vi "oa_Config Time or RPM Segment.vi"(0 "time segment":T2 {"step (s)" format="%.2f"; "end (s)" format="%.2f"; "start (s)" format="%.2f"}, 1 "plot type":T3(ring), 2 "reset in":bool, 5 "speed profile":T1 {"speed [RPM]" format="%.2f"; "time [s]" format="%.2f"}, 11 "error in (no error)":errorcluster) -> (3 "reset resampling":bool, 4 "time segment out":T2 {"step (s)" format="%.2f"; "end (s)" format="%.2f"; "start (s)" format="%.2f"}, 6 "speed profile out":T1 {"speed [RPM]" format="%.2f"; "time [s]" format="%.2f"}, 8 "reset out":bool, 10 "step found?":bool, 15 "error out":errorcluster)   [LabVIEW 2017, in "SoundVib_Resampling.lvlib"]
uses:
  <vilib>/addons/Sound and Vibration/Order Analysis/Resample Order Tracking/SoundVib_Resampling.lvlib
  <vilib>/addons/Sound and Vibration/Order Analysis/Tach Process/SubVIs/speed profile.ctl
  <vilib>/addons/Sound and Vibration/Order Analysis/Tach Process/SoundVib_TachProcess.lvlib
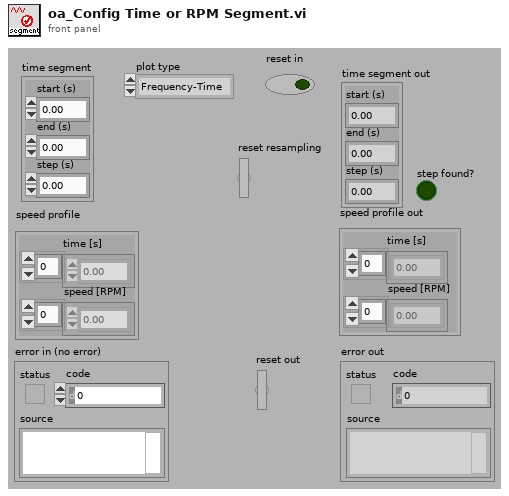
[diagram p1: front panel]
types:
  T1 = typedef "SoundVib_TachProcess.lvlib/speed profile.ctl" = cluster{"time [s]":dbl[], "speed [RPM]":dbl[]}
  T2 = cluster{"start (s)":dbl, "end (s)":dbl, "step (s)":dbl}
  T3 = enum16{"Frequency-Time", "Time-Frequency", "Order-Time", "Time-Order", "Frequency-RPM", "RPM-Frequency", "Order-RPM", "RPM-Order"}
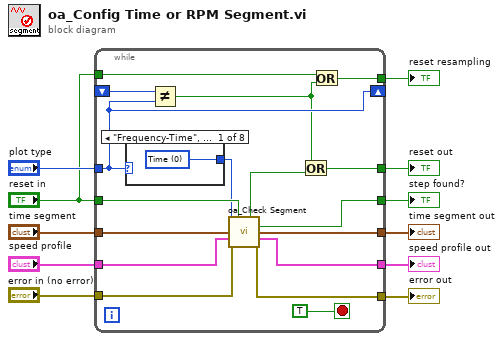
[diagram p0: block diagram]
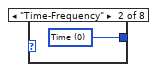
[diagram p2: hidden frame]
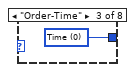
[diagram p3: hidden frame]
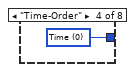
[diagram p4: hidden frame]
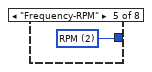
[diagram p5: hidden frame]
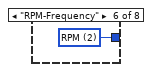
[diagram p6: hidden frame]
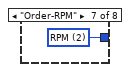
[diagram p7: hidden frame]
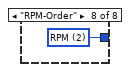
[diagram p8: hidden frame]
diagram:
  n1 = while {
    tunnel: "reset in" -> [w28]
    tunnel: "time segment" -> [w27]
    tunnel: [w26] -> w10
    tunnel: "plot type" -> [w18]
    tunnel: [w24] -> w8
    tunnel: "speed profile" -> [w23]
    tunnel: [w15] -> w6
    tunnel: "error in (no error)" -> [w22]
    tunnel: [w21] -> w4
    tunnel: [w20] -> w3
    shift-right: [w18] -> _
    shift-left: _ -> [w17]
    tunnel: "reset in" -> [w13]
    tunnel: [w12] -> w1
    stop <- TRUE stop-if-true
    n2 = case shown="\"Frequency-Time\", Default" w18 {
      tunnel: [w29 w30 w31 w32 w33 w34 w35 w36] -> w25
      frame "Frequency-Time", Default {
        w29 = u16 0 items=["Time", "Revolution", "RPM"] ("X axis selection")
      }
      frame "Time-Frequency" {
        w30 = u16 0 items=["Time", "Revolution", "RPM"] ("X axis selection")
      }
      frame "Order-Time" {
        w31 = u16 0 items=["Time", "Revolution", "RPM"] ("X axis selection")
      }
      frame "Time-Order" {
        w32 = u16 0 items=["Time", "Revolution", "RPM"] ("X axis selection")
      }
      frame "Frequency-RPM" {
        w33 = u16 2 items=["Time", "Revolution", "RPM"] ("X axis selection")
      }
      frame "RPM-Frequency" {
        w34 = u16 2 items=["Time", "Revolution", "RPM"] ("X axis selection")
      }
      frame "Order-RPM" {
        w35 = u16 2 items=["Time", "Revolution", "RPM"] ("X axis selection")
      }
      frame "RPM-Order" {
        w36 = u16 2 items=["Time", "Revolution", "RPM"] ("X axis selection")
      }
    }
    n3 = Not Equal?(x=w17, y=w18) -> (x != y?=w14:bool)
    n4 = call <vilib>:"oa_Check Segment.vi"("X axis selection"=w25, "reset?(F)"=w28, "segment position"=w27, "speed profile"=w23, "error in (no error)"=w22) -> ("reset out"=w16:bool, "step found?"=w24:bool, "segment position out"=w26:cluster{"start":dbl, "end":dbl, "step size":dbl}, "dul speed profile"=w20:T1, "error out"=w21:errorcluster)  [unwired: 5 in, 1 out]
    n5 = Or(x=w14, y=w16) -> (x .or. y?=w15:bool)
    n6 = Or(x=w13, y=w14) -> (x .or. y?=w12:bool)
  }
  "time segment out" <- w10
  "step found?" <- w8
  "error out" <- w4
  "speed profile out" <- w3
  "reset out" <- w6
  "reset resampling" <- w1
